vi "Dashboard and Primary Interface.vi"() -> ()   [LabVIEW 2023]
uses:
  C:/Users/fg/Documents/UniversalRobots.vi/UnderAutomation.UniversalRobots/lib/UnderAutomation.UniversalRobots.dll
  UnderAutomation.UniversalRobots/lib/UnderAutomation.UniversalRobots.dll
panel:
  out "Connected":bool
  out "EnumeratePrograms":string[](array[string])
  in  "Enumerate":bool
  in  "password":string
  in  "username":string
  in  "Connect SFTP":bool caption="Connect Sftp"
  in  "Program name":string
  in  "Start program":bool
  out "Powered on":bool
  in  "Script to execute":string
  in  "Send script":bool
  out "Z":dbl
  out "Y":dbl
  out "X":dbl
  in  "Robot IP":string
  out "Connect error":errorcluster
  in  "Power off":bool
  in  "Power on\nRelease brake":bool
  out "Connected":bool
  out "License state":string
  in  "Connect":bool
  # "1. Connect to the robot"
  # "2. Dashboard"
  # "3. Primary Interface"
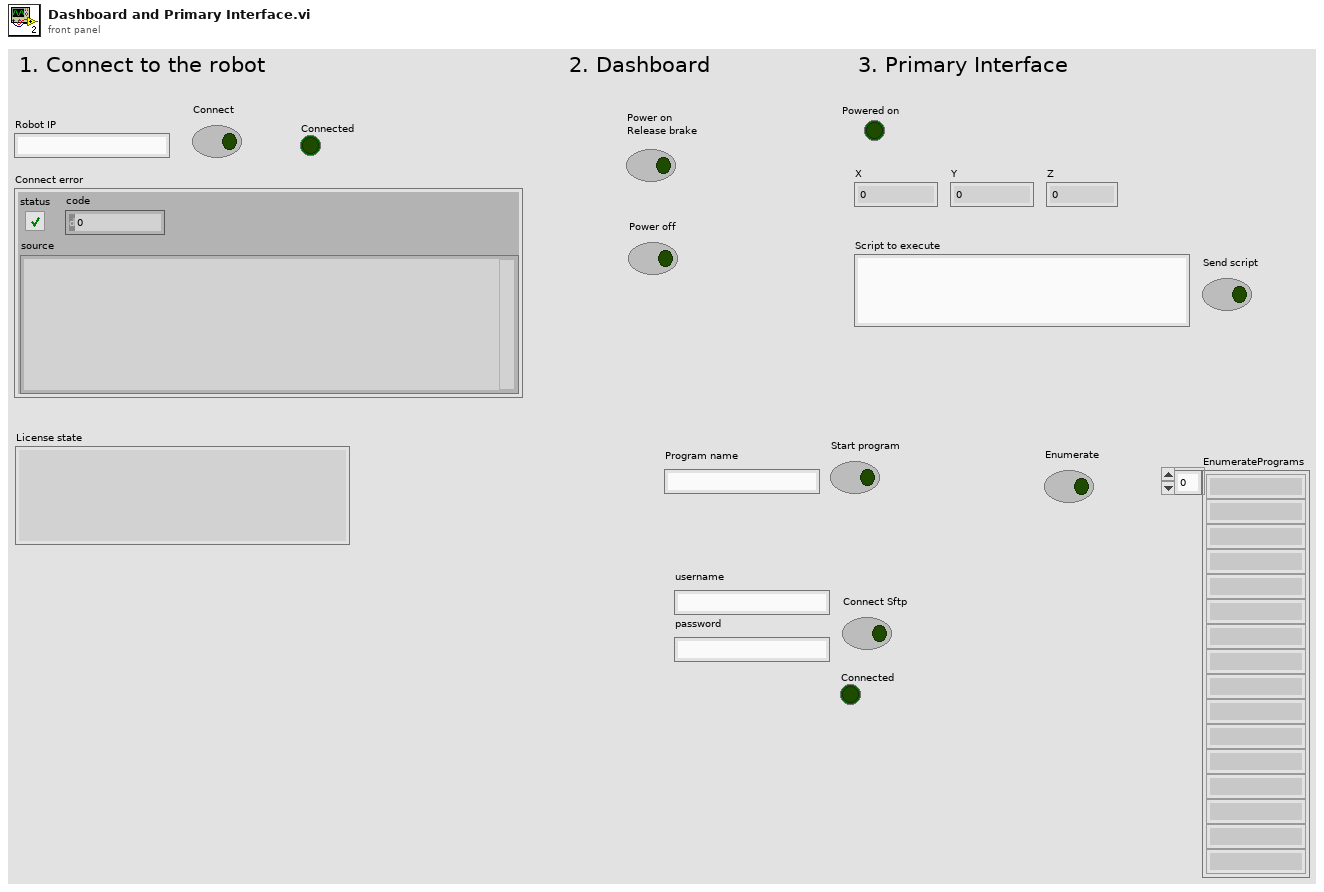
[diagram p1: front panel]
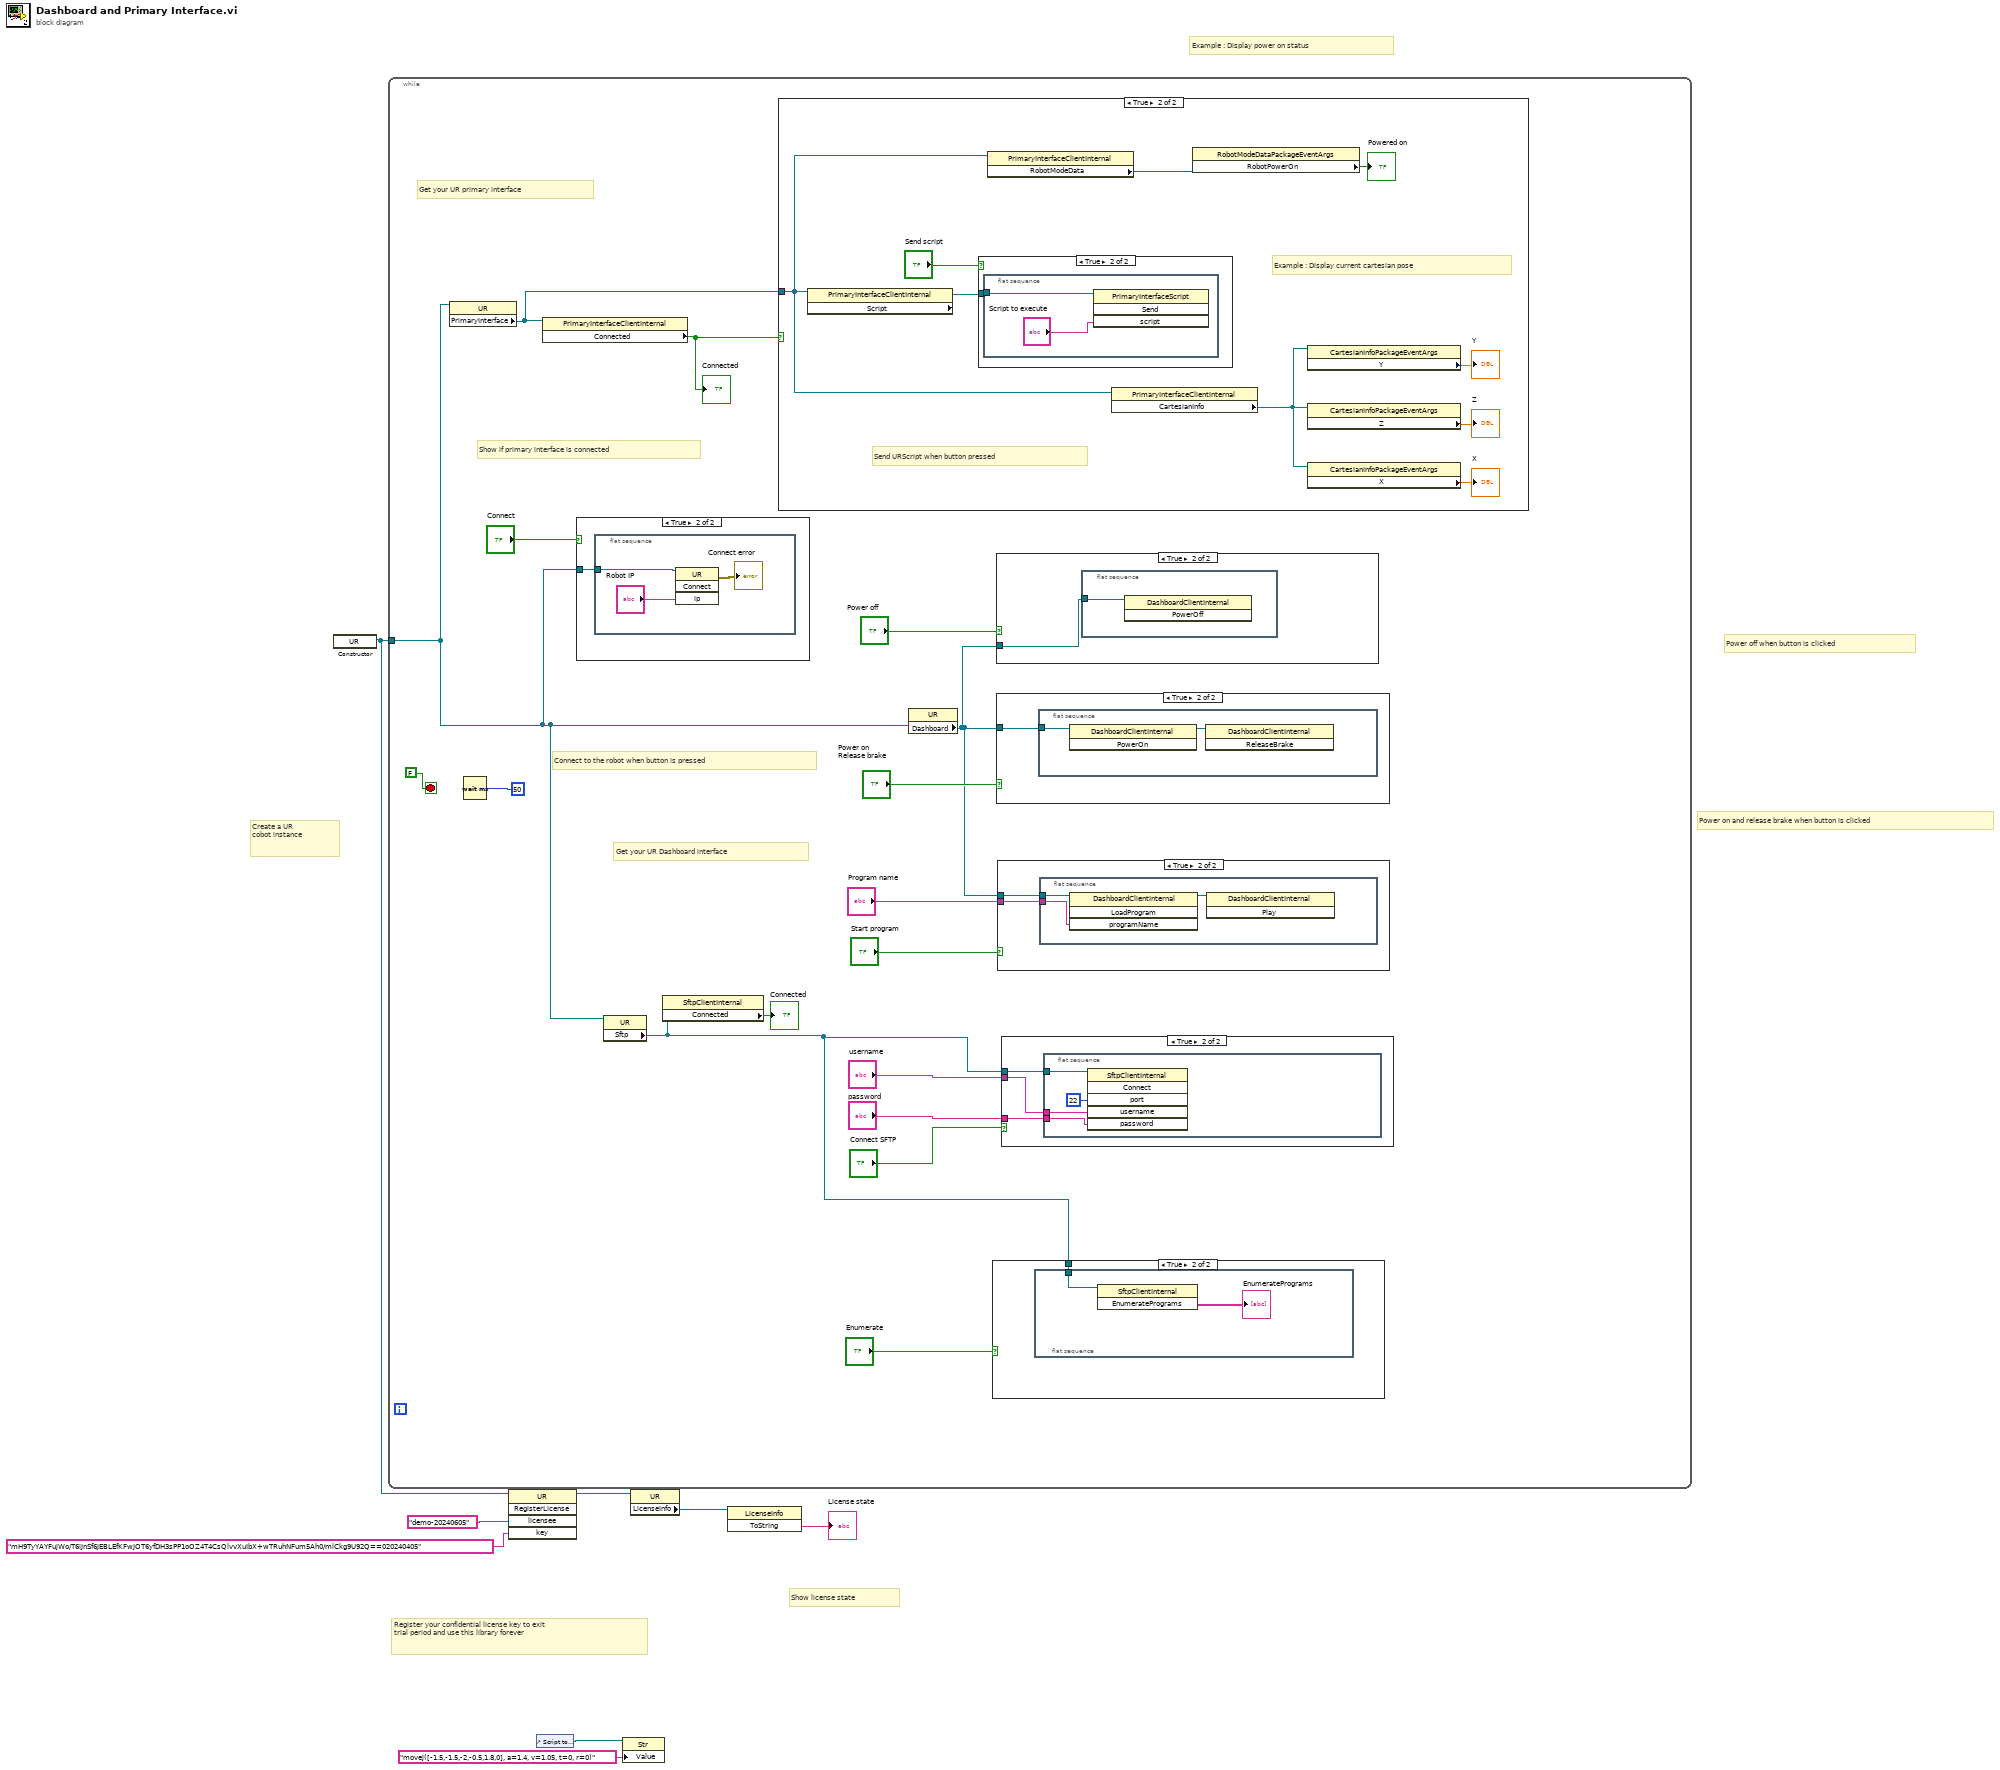
[diagram p0: block diagram]
diagram:
  # "Example : Display power on status"
  # "Create a UR\ncobot instance"
  # "Show license state"
  # "Register your confidential license key to exit\ntrial period and use this library forever"
  # "Power off when button is clicked"
  # "Power on and release brake when button is clicked"
  n1 = constructor class="UR"() -> (reference out=w3:refnum<k24>)  [unwired: 3 in, 2 out]
  n2 = while {
    tunnel: w3 -> [w15]
    stop <- FALSE stop-if-true
    # "Get your UR Dashboard interface"
    # "Connect to the robot when button is pressed"
    # "Show if primary interface is connected"
    # "Get your UR primary interface"
    n3 = property class="UR"(reference=w15) -> ("PrimaryInterface"=w21:refnum<k24>)  [unwired: 1 in, 2 out]
    n4 = Wait (ms)(milliseconds to wait=u32 50) -> ()  [unwired: 1 out]
    n5 = property class="PrimaryInterfaceClientInternal"(reference=w21) -> ("Connected"=w20:bool)  [unwired: 1 in, 2 out]
    "Connected" <- w20
    n6 = case shown="True" "Connect" {
      tunnel: w15 -> [_ w58]
      frame False {
      }
      frame True {
        n7 = flat-sequence {
          tunnel: w58 -> [w60]
          frame #0 {
            n8 = invoke class="UR" method="Connect"(reference=w60, "ip"="Robot IP") -> (error out=→"Connect error":errorcluster)  [unwired: 2 in, 3 out]
          }
        }
      }
    }
    n9 = property class="UR"(reference=w15) -> ("Sftp"=w10:refnum<k24>)  [unwired: 1 in, 2 out]
    n10 = property class="SftpClientInternal"(reference=w10) -> ("Connected"=→"Connected":bool)  [unwired: 1 in, 2 out]
    n11 = case shown="True" w20 {
      tunnel: w21 -> [_ w41]
      frame False {
      }
      frame True {
        # "Send URScript when button pressed"
        # "Example : Display current cartesian pose"
        n12 = property class="PrimaryInterfaceClientInternal"(reference=w41) -> ("Script"=w48:refnum<k24>)  [unwired: 1 in, 2 out]
        n13 = case shown="True" "Send script" {
          tunnel: w48 -> [_ w50]
          frame False {
          }
          frame True {
            n14 = flat-sequence {
              tunnel: w50 -> [w52]
              frame #0 {
                n15 = invoke class="PrimaryInterfaceScript" method="Send"(reference=w52, "script"="Script to execute") -> ()  [unwired: 2 in, 4 out]
              }
            }
          }
        }
        n16 = property class="PrimaryInterfaceClientInternal"(reference=w41) -> ("RobotModeData"=w47:refnum<k24>)  [unwired: 1 in, 2 out]
        n17 = property class="PrimaryInterfaceClientInternal"(reference=w41) -> ("CartesianInfo"=w42:refnum<k24>)  [unwired: 1 in, 2 out]
        n18 = property class="RobotModeDataPackageEventArgs"(reference=w47) -> ("RobotPowerOn"=→"Powered on":bool)  [unwired: 1 in, 2 out]
        n19 = property class="CartesianInfoPackageEventArgs"(reference=w42) -> ("Y"=→"Y":dbl)  [unwired: 1 in, 2 out]
        n20 = property class="CartesianInfoPackageEventArgs"(reference=w42) -> ("Z"=→"Z":dbl)  [unwired: 1 in, 2 out]
        n21 = property class="CartesianInfoPackageEventArgs"(reference=w42) -> ("X"=→"X":dbl)  [unwired: 1 in, 2 out]
      }
    }
    n22 = property class="UR"(reference=w15) -> ("Dashboard"=w17:refnum<k24>)  [unwired: 1 in, 2 out]
    n23 = case shown="True" "Enumerate" {
      tunnel: w10 -> [_ w26]
      frame False {
      }
      frame True {
        n24 = flat-sequence {
          tunnel: w26 -> [w28]
          frame #0 {
            n25 = invoke class="SftpClientInternal" method="EnumeratePrograms"(reference=w28) -> ("EnumeratePrograms"=→"EnumeratePrograms":string[])  [unwired: 2 in, 2 out]
          }
        }
      }
    }
    n26 = case shown="True" "Power off" {
      tunnel: w17 -> [_ w53]
      frame False {
      }
      frame True {
        n27 = flat-sequence {
          tunnel: w53 -> [w54]
          frame #0 {
            n28 = invoke class="DashboardClientInternal" method="PowerOff"(reference=w54) -> ()  [unwired: 2 in, 3 out]
          }
        }
      }
    }
    n29 = case shown="True" "Power on\nRelease brake" {
      tunnel: w17 -> [_ w55]
      frame False {
      }
      frame True {
        n30 = flat-sequence {
          tunnel: w55 -> [w57]
          frame #0 {
            n31 = invoke class="DashboardClientInternal" method="PowerOn"(reference=w57) -> (reference out=w56:refnum<k24>)  [unwired: 2 in, 2 out]
            n32 = invoke class="DashboardClientInternal" method="ReleaseBrake"(reference=w56) -> ()  [unwired: 2 in, 3 out]
          }
        }
      }
    }
    n33 = case shown="True" "Start program" {
      tunnel: w17 -> [_ w37]
      tunnel: "Program name" -> [_ w36]
      frame False {
      }
      frame True {
        n34 = flat-sequence {
          tunnel: w37 -> [w40]
          tunnel: w36 -> [w38]
          frame #0 {
            n35 = invoke class="DashboardClientInternal" method="LoadProgram"(reference=w40, "programName"=w38) -> (reference out=w39:refnum<k24>)  [unwired: 2 in, 3 out]
            n36 = invoke class="DashboardClientInternal" method="Play"(reference=w39) -> ()  [unwired: 2 in, 3 out]
          }
        }
      }
    }
    n37 = case shown="True" "Connect SFTP" {
      tunnel: w10 -> [_ w31]
      tunnel: "username" -> [_ w30]
      tunnel: "password" -> [_ w29]
      frame False {
      }
      frame True {
        n38 = flat-sequence {
          tunnel: w31 -> [w35]
          tunnel: w30 -> [w33]
          tunnel: w29 -> [w34]
          frame #0 {
            n39 = invoke class="SftpClientInternal" method="Connect"(reference=w35, "port"=22, "username"=w33, "password"=w34) -> ()  [unwired: 2 in, 6 out]
          }
        }
      }
    }
  }
  n40 = invoke class="UR" method="RegisterLicense"(reference=w3, "licensee"="demo-20240605", "key"="mH9TyYAYFujWo/T6iJnSf6JEBLEfKFwJOT6yfDH3sPP1oOZ4T4CsQlvvXuIbX+wTRuhNFum5Ah0/mlCkg9U92Q==020240405") -> (reference out=w5:refnum<k24>)  [unwired: 2 in, 4 out]
  n41 = control-ref of="Script to execute"() -> (w2:refnum<vi>)
  n42 = property class="Str"(reference=w2, "Value"="movej([-1.5,-1.5,-2,-0.5,1.8,0], a=1.4, v=1.05, t=0, r=0)") -> ()  [unwired: 1 in, 2 out]
  n43 = property class="UR"(reference=w5) -> ("LicenseInfo"=w4:refnum<k24>)  [unwired: 1 in, 2 out]
  n44 = invoke class="LicenseInfo" method="ToString"(reference=w4) -> ("ToString"=→"License state":string)  [unwired: 2 in, 2 out]
